vi "Read Loop.vi"(8 "error in (no error)":errorcluster, 9 "ReadElements":u32, 10 "Queues":T1, 11 "AODAcq in":refnum<class "AODAcq.lvclass">) -> (0 "error out":errorcluster, 2 "Done":bool=TRUE, 3 "AODAcq out":refnum<class "AODAcq.lvclass">)   [LabVIEW 2011, in "AODAcq.lvclass"]
uses:
  AODAcq.lvclass
panel:
  out "Progress":dbl(slide) scale=0.0..1.0
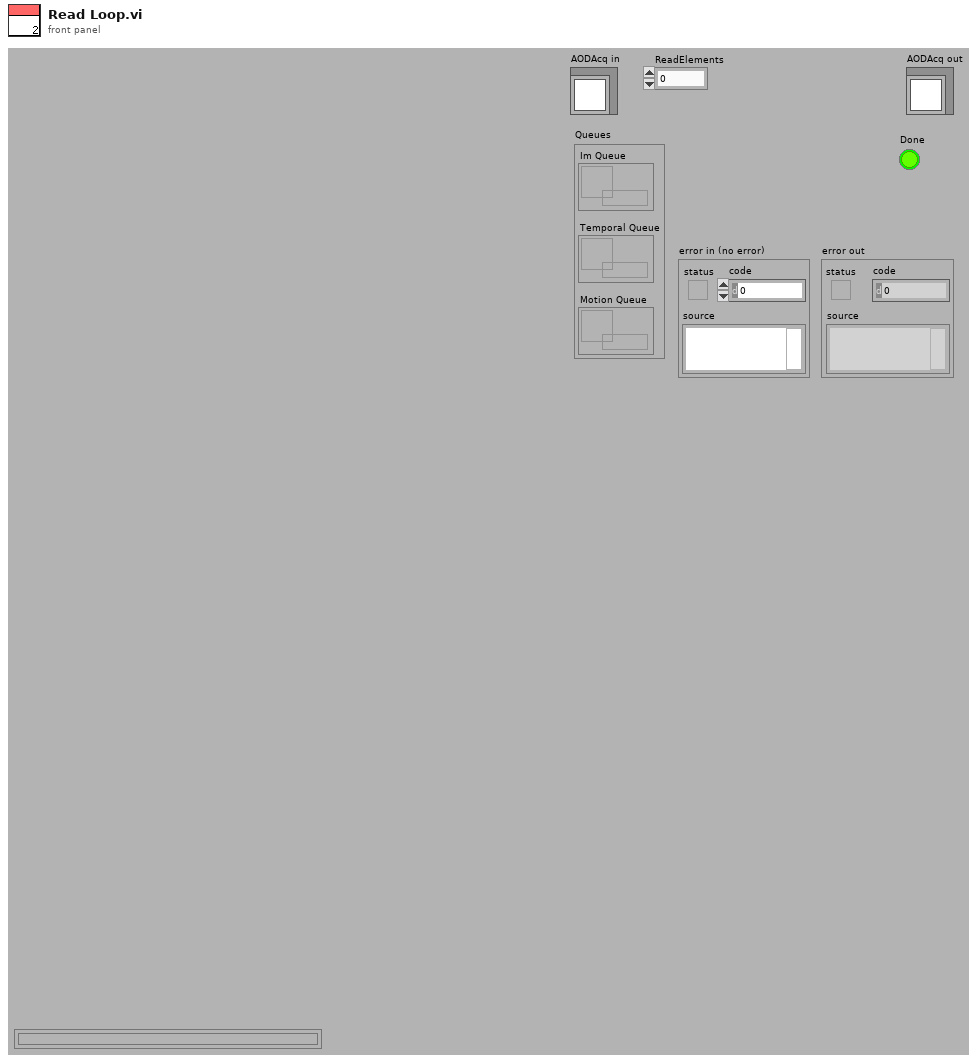
[diagram p1: front panel]
types:
  T1 = cluster{"Im Queue":refnum<queue>, "Temporal Queue":refnum<queue>, "Motion Queue":refnum<queue>}
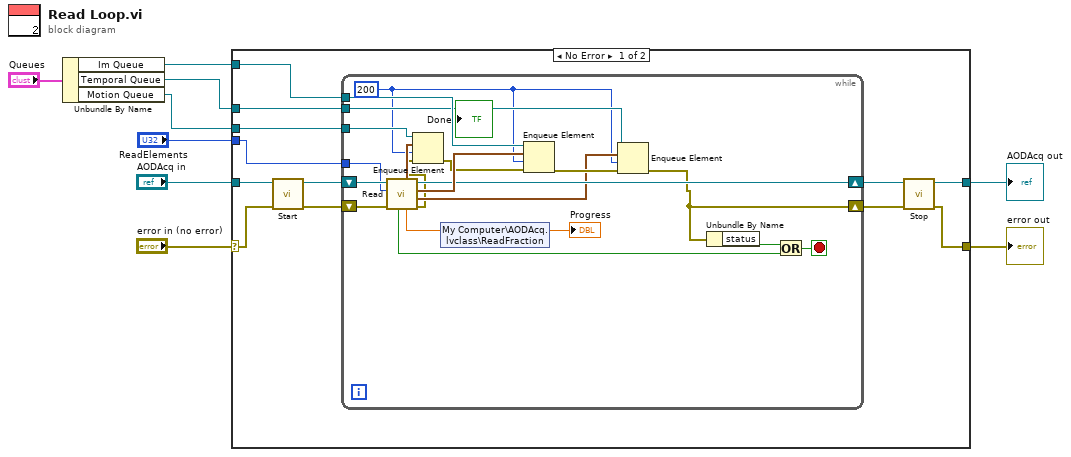
[diagram p0: block diagram]
diagram:
  n1 = Unbundle By Name("Queues") -> ("Im Queue"=w3:refnum<queue>, "Temporal Queue"=w2:refnum<queue>, "Motion Queue"=w1:refnum<queue>)
  n2 = case shown="No Error" "error in (no error)" {
    selector: "error in (no error)" -> [w16 w42]
    tunnel: [w14 w42] -> w8
    tunnel: [w17 w41] -> w6
    tunnel: "AODAcq in" -> [w19 w41]
    tunnel: w3 -> [w13 _]
    tunnel: "ReadElements" -> [w12 _]
    tunnel: w2 -> [w11 _]
    tunnel: w1 -> [w10 _]
    frame No Error {
      n3 = call-dynamic "Start.vi"("error in (no error)"=w16, "AODAcq in"=w19) -> ("error out"=w20:errorcluster, "AODAcq out"=w21:refnum<class "AODAcq.lvclass">)  [unwired: 8 in]
      n4 = while {
        tunnel: w13 -> [w38]
        tunnel: w12 -> [w35]
        shift-right: [w32] -> w18
        shift-left: w21 -> [w40]
        shift-right: [w22] -> w15
        shift-left: w20 -> [w39]
        tunnel: w11 -> [w28]
        tunnel: w10 -> [w26]
        stop <- w33 stop-if-true
        w23 = 200 ("timeout in ms (-1)")
        n5 = call-dynamic "Read.vi"("error in (no error)"=w39, "ReadElements"=w35, "AODAcq in"=w40) -> ("error out"=w25:errorcluster, "TemporalData"=w29:waveform(dbl)[], "ImData"=w37:waveform(i32)[], "AODAcq out"=w32:refnum<class "AODAcq.lvclass">, "ReadFraction"=w36:dbl, "MotionData"=w27:waveform(i32)[], "Done"=w31:bool)  [unwired: 2 in]
        "Progress" <- w36
        n6 = Enqueue Element(queue=w26, element=w27, timeout in ms (-1)=w23, error in (no error)=w25) -> (error out=w24:errorcluster)  [unwired: 2 out]
        n7 = shared-variable "My Computer\\AODAcq.lvclass\\ReadFraction"(w36) -> ()  [unwired: 1 in, 1 out]
        n8 = Enqueue Element(queue=w38, element=w37, timeout in ms (-1)=w23, error in (no error)=w24) -> (error out=w30:errorcluster)  [unwired: 2 out]
        n9 = Enqueue Element(queue=w28, element=w29, timeout in ms (-1)=w23, error in (no error)=w30) -> (error out=w22:errorcluster)  [unwired: 2 out]
        n10 = Unbundle By Name(w22) -> ("status"=w34:bool)
        n11 = Or(x=w34, y=w31) -> (x .or. y?=w33:bool)
      }
      n12 = call-dynamic "Stop.vi"("error in (no error)"=w15, "AODAcq in"=w18) -> ("error out"=w14:errorcluster, "AODAcq out"=w17:refnum<class "AODAcq.lvclass">)  [unwired: 8 in]
    }
    frame Error {
    }
  }
  "error out" <- w8
  "AODAcq out" <- w6
